vi "Examples - AcquisitionTest.vi"() -> ()   [LabVIEW 2015]
panel:
  in  "Stop":bool
  out "Image":T1(plugin-control)
  # "Use this button instead of Abort Execution button"
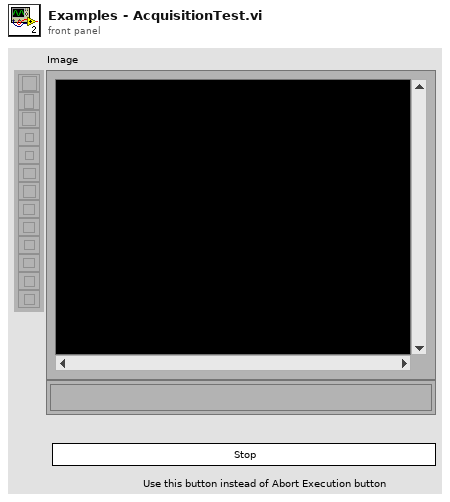
[diagram p1: front panel]
types:
  T1 = typedef "IMAQ Image.ctl" = refnum<image>
  T2 = typedef "Image Type" = u32
  T3 = typedef "xiImageMng - Attributes.ctl" = cluster{"WIDTH":i32, "HEIGHT":i32, "IMG_FORMAT":T4}
  T4 = typedef "IMG_DATA_FORMAT.ctl" = enum16{"MONO8", "MONO16", "RGB24", "RGB32", "RGBPLANAR", "RAW8", "RAW16"}
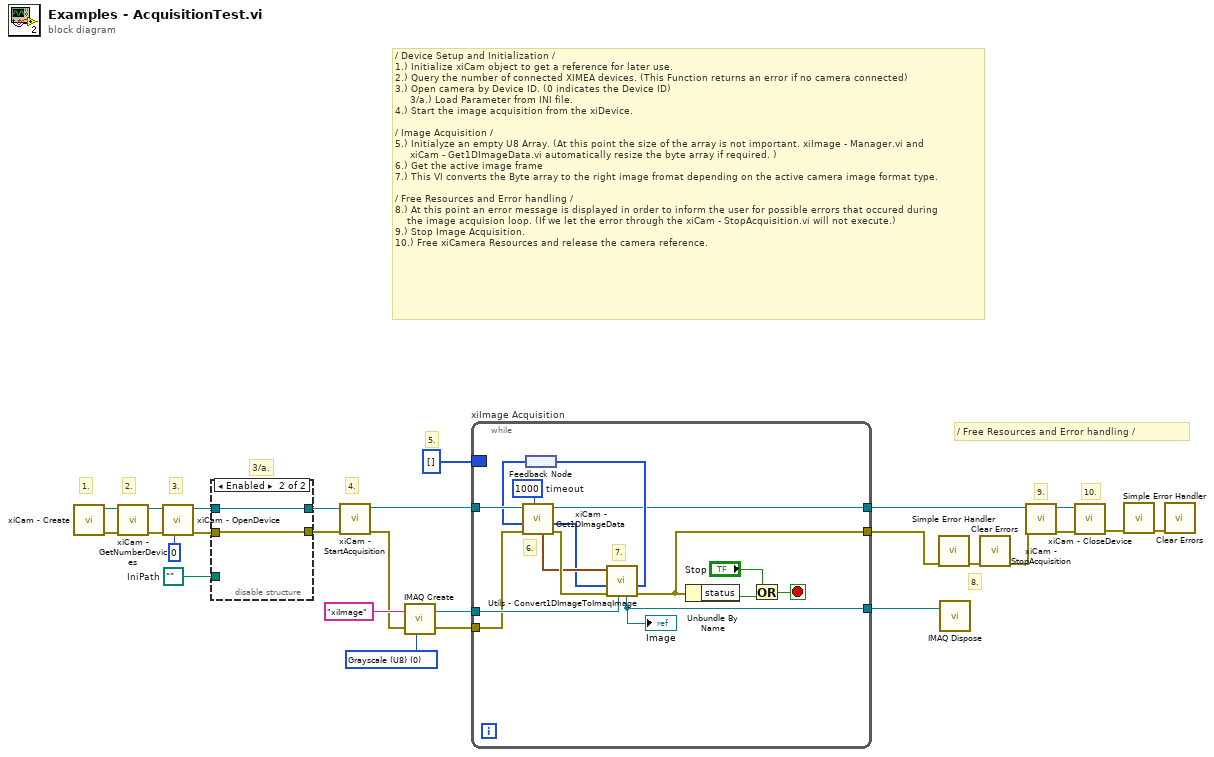
[diagram p0: block diagram]
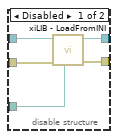
[diagram p2: hidden frame]
diagram:
  w3 = T2 0 items=["Grayscale (U8)", "Grayscale (I16)", "Grayscale (SGL)", "Complex (CSG)", "RGB (U32)", "HSL (U32)", "RGB (U64)", "Grayscale (U16)"] ("Image Type")
  w4 = path ""  # IniPath
  # "3/a."
  # "/ Free Resources and Error handling /"
  # "9."
  # "10."
  # "8."
  # "5."
  # "/ Device Setup and Initialization /\n1.) Initialize xiCam object to get a reference for later use.\n2.) Query the number of connected XIMEA devices. (This Function returns an error if no camera connected)\n3.) Open camera by Device ID. (0 indicates the Device ID)\n     3/a.) Load Parameter from INI file. \n4.) Start the image acquisition from the xiDevice.\n\n/ Image Acquisition /\n5.) Initialyze an empty U8 Array. (At this point the size of the array is not important. xiImage - Manager.vi and\n     xiCam - Get1DImageData.vi automatically resize the byte array if required. )\n6.) Get the active image frame\n7.) This VI converts the Byte array to the right image fromat depending on the active camera image format type.\n\n/ Free Resources and Error handling /\n8.) At this point an error message is displayed in order to inform the user for possible errors that occured during\n    the image acquision loop. (If we let the error through the xiCam - StopAcquisition.vi will not execute.)\n9.) Stop Image Acquisition.\n10.) Free xiCamera Resources and release the camera reference."
  # "4."
  # "3."
  # "2."
  # "1."
  n1 = call "xiCam - Create.vi"() -> ("error out"=w25:errorcluster, "new xiCam"=w26:refnum<k24>)  [unwired: 10 in]
  n2 = call "xiCam - GetNumberDevices.vi"("error in (no error)"=w25, "xiCam In"=w26) -> ("error out"=w23:errorcluster, "xiCam Out"=w24:refnum<k24>)  [unwired: 7 in, 1 out]
  n3 = call "xiCam - OpenDevice.vi"("DevID"=0, "error in (no error)"=w23, "xiCam In"=w24) -> ("error out"=w5:errorcluster, "xiCam Out"=w6:refnum<k24>)  [unwired: 7 in]
  n4 = disable-structure shown="Enabled" {
    disable-tunnel: w6 -> [w31 w33]
    disable-tunnel: [w30 w33] -> w2
    disable-tunnel: [w29 w32] -> w1
    disable-tunnel: w5 -> [w28 w32]
    disable-tunnel: w4 -> [w27 _]
    frame Disabled {
      n5 = call "xiLIB - LoadFromINI.vi"("IniPath"=w27, "Error In"=w28, "xiCam In"=w31) -> ("Error Out"=w29:errorcluster, "xiCam Out"=w30:refnum<k24>)  [unwired: 7 in]
    }
    frame Enabled {
    }
  }
  n6 = call "xiCam - StartAcquisition.vi"("error in (no error)"=w1, "xiCam In"=w2) -> ("error out"=w9:errorcluster, "xiCam Out"=w21:refnum<k24>)  [unwired: 8 in]
  n7 = call "IMAQ Create"("Image Name"="xiImage", "Image Type"=w3, "error in (no error)"=w9) -> ("New Image"=w10:T1, "error out"=w8:errorcluster)  [unwired: 2 in]
  n8 = while "xiImage Acquisition" {
    tunnel: w21 -> [w48]
    border: u8[] [] ("1DImageData Out") -> [_]
    tunnel: [w38] -> w18
    tunnel: [w37] -> w19
    tunnel: w10 -> [w36]
    tunnel: w8 -> [w35]
    tunnel: [w34] -> w7
    stop <- w39 stop-if-true
    w46 = 1000  # timeout
    # "7."
    # "6."
    n9 = feedback #1() -> (w47:u8[])
    n10 = call "xiCam - Get1DImageData.vi"("timeout"=w46, "error in (no error)"=w35, "1DImageData In"=w47, "xiCam In"=w48) -> ("error out"=w45:errorcluster, "1DImageData Out"=w43:u8[], "xiCam Out"=w37:refnum<k24>, "Image Properites"=w44:T3)  [unwired: 4 in]
    n11 = call "Utils - Convert1DImageToImaqImage.vi"("Image In"=w36, "error in (no error)"=w45, "1DImageData In"=w43, "Image Properties In"=w44) -> ("error out"=w38:errorcluster, "1DImageData Out"=w42:u8[], "Image Out"=w34:T1)  [unwired: 5 in]
    "Image" <- w34
    n12 = feedback-in #1(w42) -> ()
    n13 = Unbundle By Name(w38) -> ("status"=w41:bool)
    n14 = Or(x="Stop", y=w41) -> (x .or. y?=w39:bool)
  }
  n15 = call <vilib>:"Simple Error Handler.vi"("error in (no error)"=w18) -> ("error out"=w17:errorcluster)  [unwired: 4 in, 4 out]
  n16 = call "IMAQ Dispose"("Image"=w7) -> ()  [unwired: 5 in, 1 out]
  n17 = call <vilib>:"Clear Errors.vi"("error in (no error)"=w17) -> ("error out"=w16:errorcluster)  [unwired: 5 in, 1 out]
  n18 = call "xiCam - StopAcquisition.vi"("error in (no error)"=w16, "xiCam In"=w19) -> ("error out"=w14:errorcluster, "xiCam Out"=w15:refnum<k24>)  [unwired: 8 in]
  n19 = call "xiCam - CloseDevice.vi"("error in (no error)"=w14, "xiCam In"=w15) -> ("error out"=w12:errorcluster)  [unwired: 9 in]
  n20 = call <vilib>:"Simple Error Handler.vi"("error in (no error)"=w12) -> ("error out"=w13:errorcluster)  [unwired: 4 in, 4 out]
  n21 = call <vilib>:"Clear Errors.vi"("error in (no error)"=w13) -> ()  [unwired: 5 in, 2 out]
